vi "Add Message Buffer (RT).vi"(6 "MessageData (0x0000)":u16[](array[numeric]) format="%04x", 8 "error in":errorcluster, 9 "MessageBuffer configuration":T1={"bufferMaxEntries"=1, "bufferType"=0, "eventLogOnEmptyOrFull"=FALSE, "eventLogOnHalf"=FALSE} {"bufferType" items=["FIFO", "Circular"]}, 10 "name":string="CoreName", 11 "Remote Terminal in":refnum<k24>) -> (0 "error out":errorcluster, 1 "ID out":i32, 2 "new messageBuffer":refnum<k24>, 3 "Remote Terminal out":refnum<k24>)   [LabVIEW 2020, in "Ballard_1553_Hardware_ni.lvlib"]
uses:
  Ballard_1553_Hardware_ni.lvlib
  C:/Users/Administrator/Desktop/GIT/Ballard-MIL-STD-1553-Custom-Device/Source/System Explorer/SubVIs/Parse XML Ballard/1.2/BTIXML_SerDes.dll
  Ballard-MIL-STD-1553-Custom-Device/Source/System Explorer/SubVIs/Parse XML Ballard/1.2/BTIXML_SerDes.dll
  _typedefs/MessageBuffer_type.ctl
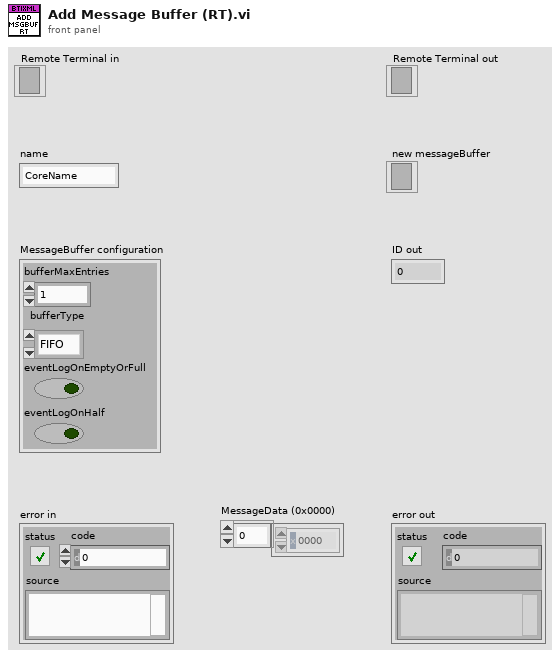
[diagram p1: front panel]
types:
  T1 = typedef "Ballard_1553_Hardware_ni.lvlib/MessageBuffer_type.ctl" = cluster{"bufferMaxEntries":i32, "bufferType":i32, "eventLogOnEmptyOrFull":bool, "eventLogOnHalf":bool}
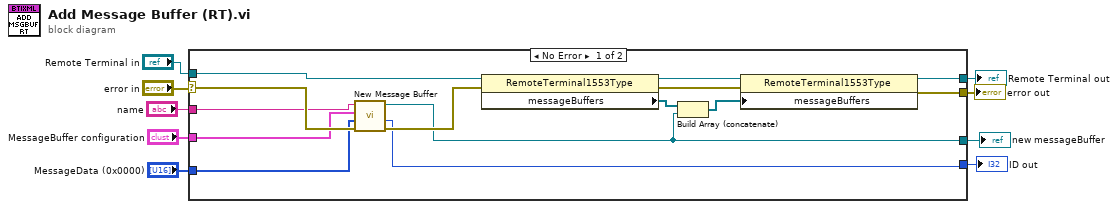
[diagram p0: block diagram]
diagram:
  n1 = case shown="No Error" "error in" {
    selector: "error in" -> [w17 w24]
    tunnel: [w21 w24] -> w9
    tunnel: [w22 w25] -> w8
    tunnel: "Remote Terminal in" -> [w23 w25]
    tunnel: "name" -> [w15 _]
    tunnel: "MessageBuffer configuration" -> [w14 _]
    tunnel: "MessageData (0x0000)" -> [w13 _]
    tunnel: [w12 _] -> w1
    tunnel: [w11 _] -> w2
    frame No Error {
      n2 = call "New Message Buffer.vi"("error in"=w17, "MessageData (0x0000)"=w13, "MessageBuffer configuration"=w14, "name"=w15) -> ("error out"=w16:errorcluster, "ID out"=w12:i32, "new messageBuffer"=w11:refnum<k24>)  [unwired: 5 in]
      n3 = property class="RemoteTerminal1553Type"(reference=w23, error in=w16) -> (reference out=w19:refnum<k24>, error out=w20:errorcluster, "messageBuffers"=w18:refnum<k24>[])
      n4 = Build Array (concatenate)(w18, w11) -> (w10:refnum<k24>[])
      n5 = property class="RemoteTerminal1553Type"(reference=w19, error in=w20, "messageBuffers"=w10) -> (reference out=w22:refnum<k24>, error out=w21:errorcluster)
    }
    frame Error {
    }
  }
  "error out" <- w9
  "Remote Terminal out" <- w8
  "new messageBuffer" <- w2
  "ID out" <- w1
